vi "FeedbackDecode_UpdateDatabase.vi"(3 "DatabaseIn":T1={"ExperimentDate"=timestamp(3401556199.892892 s since 1904-01-01), "ImplantDate"=timestamp(3401890063 s since 1904-01-01), "CerebusFolder"="", "Experimenter"="Tyler Davis", "PatientNumber"="201102", "DominantHand"="Right", "DeviceType"="uECOG", "DeviceSerial"="CG-64BPX-F419", "DeviceHemisphere"="Right", "DeviceRegion"="Hand", "TaskType"="ArmMovementTask.vi", "TaskComments"="", "RecordingComments"="", "GeneralObservations"=""}, 4 "RecordsSelection":string="10/16/2011\u0000\u0000\u0000\u0000\u0000\u0000\u0000\u0000\u0000\u0000\u0000\u0000", 5 "CallType":enum16{"Initialize", "Save", "Load"}(ring)=enum."Load", 6 "DatabaseUDL":path=path "E:/Data/PatientDatabase.udl") -> (0 "DatabaseOut":T1={"ExperimentDate"=timestamp(3401556199.892892 s since 1904-01-01), "ImplantDate"=timestamp(3401890063 s since 1904-01-01), "CerebusFolder"="", "Experimenter"="Tyler Davis", "PatientNumber"="201102", "DominantHand"="Right", "DeviceType"="uECOG", "DeviceSerial"="CG-64BPX-F419", "DeviceHemisphere"="Right", "DeviceRegion"="Hand", "TaskType"="ArmMovementTask.vi", "TaskComments"="", "RecordingComments"="", "GeneralObservations"=""}, 1 "CerebusFoldersDates":string[](array[string]), 2 "ExperimentDatesSorted":string[](array[string]))   [LabVIEW 2020]
uses:
  <vilib>/addons/database/Connection.llb/DB Tools Open Connec (Path).vi
  <vilib>/addons/database/_DB Variant To Data/Database Variant To Data.xnode
  <vilib>/addons/database/NI_Database_API.lvlib
panel:
  out "ExperimentDates":string[](array[string])
  out "Fields":string[](array[string])=["ExperimentDate", "ImplantDate", "CerebusFolder", "Experimenter", "PatientNumber", "DominantHand", "DeviceType", "DeviceSerial", "DeviceHemisphere", "DeviceRegion", "TaskType", "TaskComments", "RecordingComments", "GeneralObservations"]
  # "Do not place ';' or '=' in the comment fields"
  # "Do not place ';' or '=' in the comment fields"
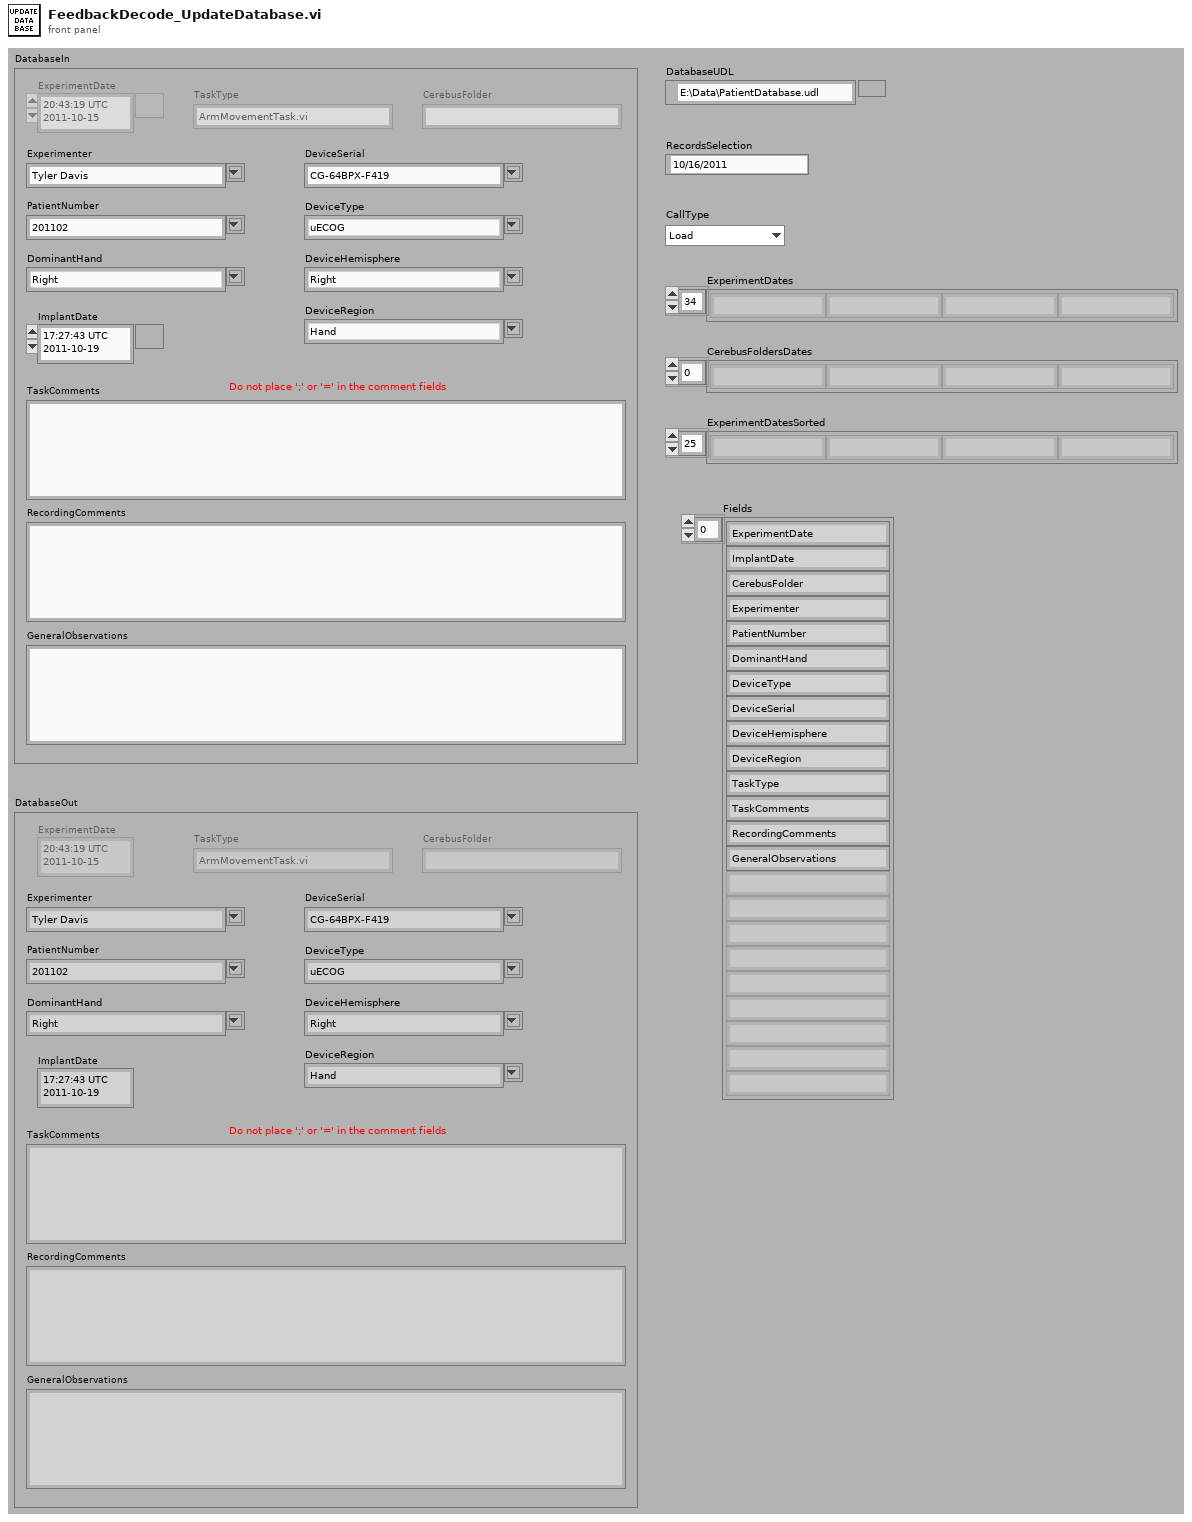
[diagram p1: front panel]
types:
  T1 = cluster{"ExperimentDate":timestamp, "ImplantDate":timestamp, "CerebusFolder":string, "Experimenter":string, "PatientNumber":string, "DominantHand":string, "DeviceType":string, "DeviceSerial":string, "DeviceHemisphere":string, "DeviceRegion":string, "TaskType":string, "TaskComments":string, "RecordingComments":string, "GeneralObservations":string}
  T2 = typedef "NI_Database_API.lvlib/Conn ObjectReference.ctl" = refnum<k1>
  T3 = cluster{"data":timestamp, "data":timestamp, "data":string, "data":string, "data":string, "data":string, "data":string, "data":string, "data":string, "data":string, "data":string, "data":string, "data":string, "data":string}
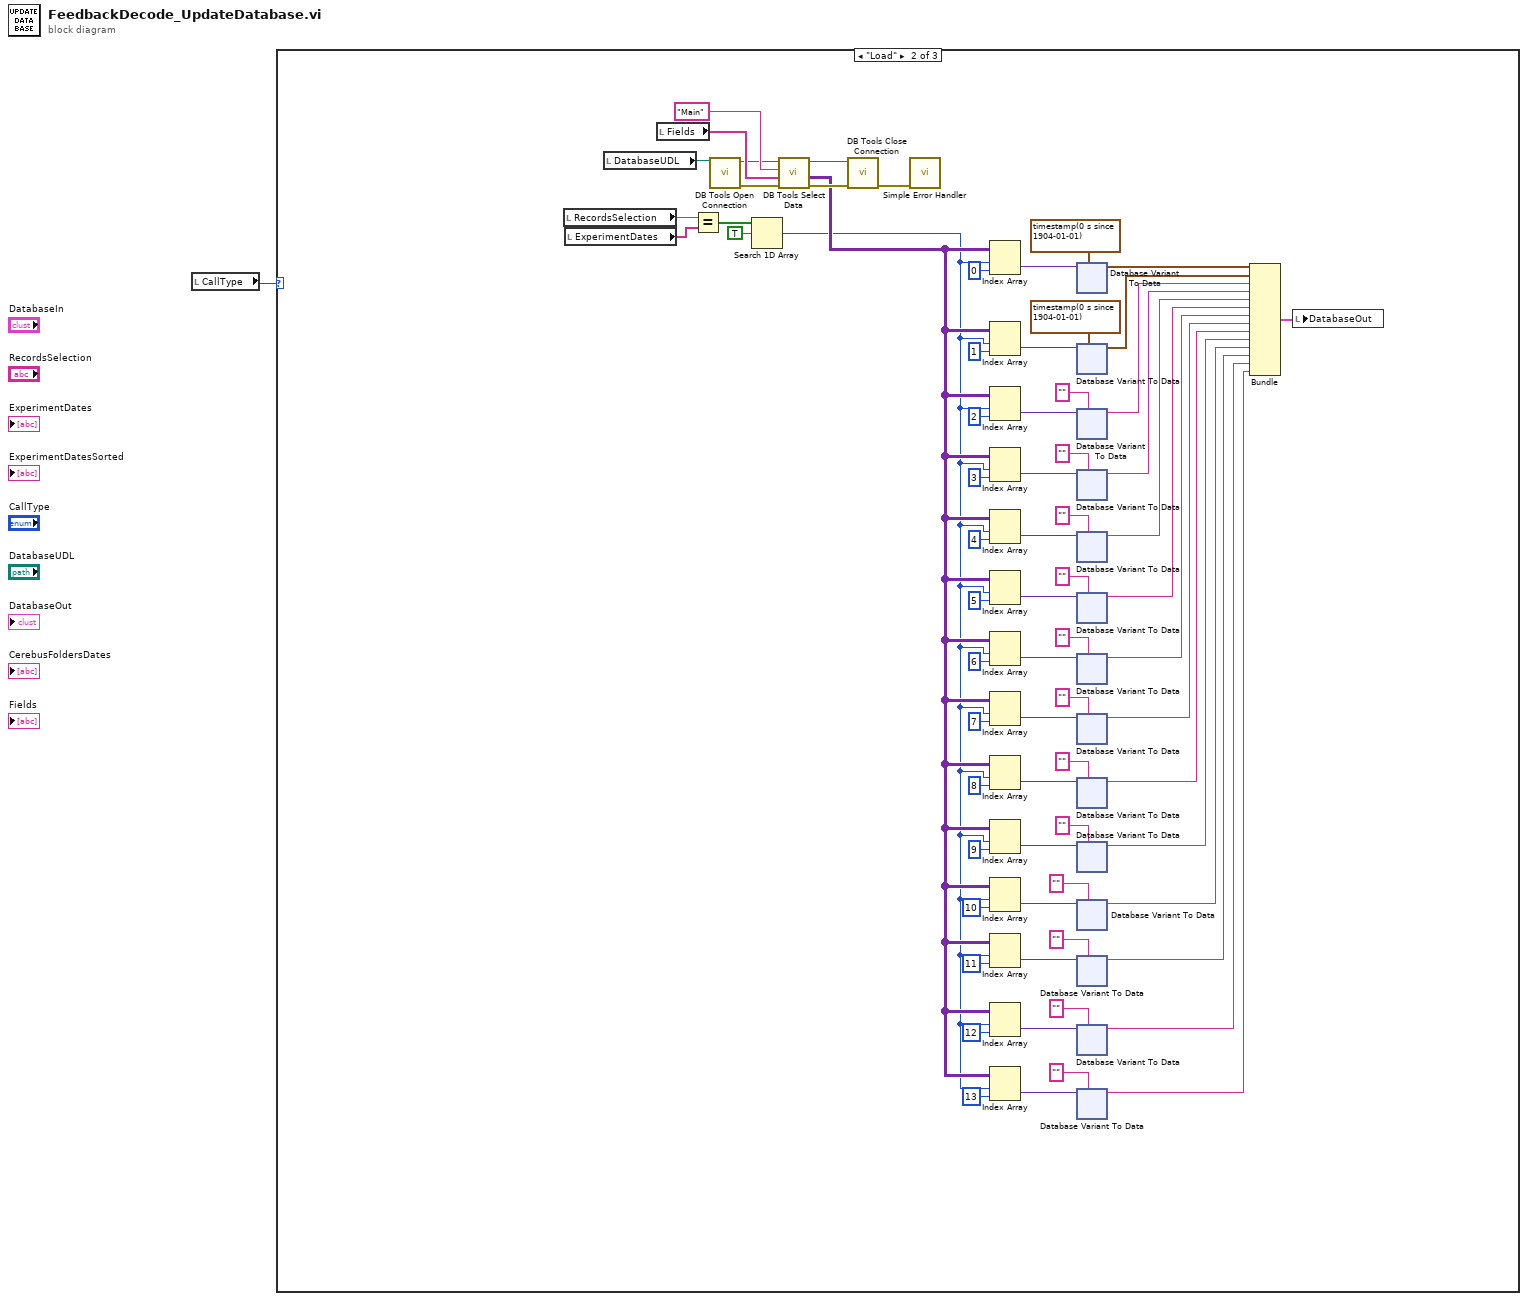
[diagram p0: block diagram]
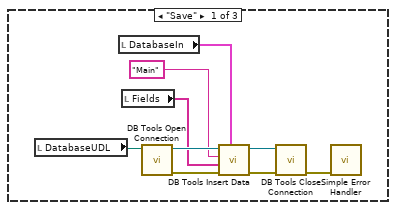
[diagram p2: hidden frame]
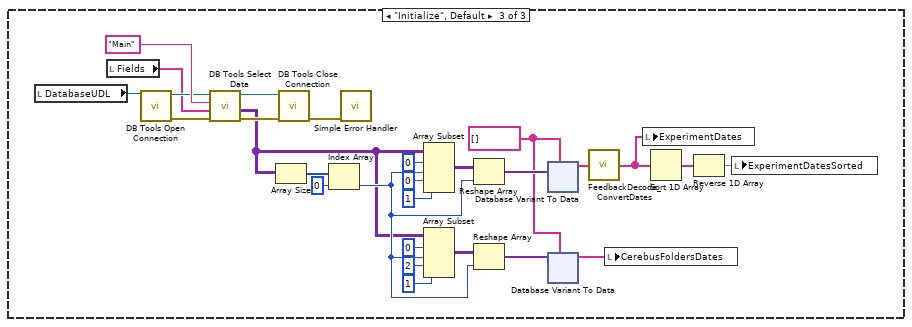
[diagram p3: hidden frame]
diagram:
  n1 = local read "CallType"() -> (w1:enum16{"Initialize", "Save", "Load"})
  n2 = case shown="\"Load\"" w1 {
    frame "Save" {
      n3 = local read "DatabaseUDL"() -> (w2:path)
      n4 = local read "DatabaseIn"() -> (w3:T1)
      n5 = local read "Fields"() -> (w4:string[])
      n6 = call-poly <vilib>:"DB Tools Open Connection.vi"("connection information"=w2) -> ("error out"=w8:errorcluster, "connection reference"=w10:T2)  [unwired: 7 in]
      n7 = call <vilib>:"DB Tools Insert Data.vi"("data"=w3, "error in (no error)"=w8, "columns"=w4, "table"="Main", "connection reference"=w10) -> ("error out"=w7:errorcluster, "connection reference out"=w6:T2)  [unwired: 5 in]
      n8 = call <vilib>:"DB Tools Close Connection.vi"("error in (no error)"=w7, "connection reference"=w6) -> ("error out"=w5:errorcluster)  [unwired: 5 in]
      n9 = call <vilib>:"Simple Error Handler.vi"("error in (no error)"=w5) -> ()  [unwired: 4 in, 5 out]
    }
    frame "Load" {
      n10 = local read "RecordsSelection"() -> (w32:string)
      n11 = local read "ExperimentDates"() -> (w31:string[])
      n12 = local read "DatabaseUDL"() -> (w79:path)
      n13 = local read "Fields"() -> (w77:string[])
      n14 = Equal?(x=w32, y=w31) -> (x = y?=w33:bool[])
      n15 = call-poly <vilib>:"DB Tools Open Connection.vi"("connection information"=w79) -> ("error out"=w81:errorcluster, "connection reference"=w74:T2)  [unwired: 7 in]
      n16 = Search 1D Array(1D array=w33, element=TRUE) -> (index of element=w11:i32)  [unwired: 1 in]
      n17 = call <vilib>:"DB Tools Select Data.vi"("error in (no error)"=w81, "columns"=w77, "table"="Main", "connection reference"=w74) -> ("error out"=w76:errorcluster, "data"=w13:variant[][], "connection reference out"=w75:T2)  [unwired: 2 in]
      n18 = call <vilib>:"DB Tools Close Connection.vi"("error in (no error)"=w76, "connection reference"=w75) -> ("error out"=w80:errorcluster)  [unwired: 5 in]
      n19 = call <vilib>:"Simple Error Handler.vi"("error in (no error)"=w80) -> ()  [unwired: 4 in, 5 out]
      n20 = Index Array(array=w13, index (row)=w11, index (col)=0 ("disabled index (col)")) -> (element=w72:variant)
      n21 = Index Array(array=w13, index (row)=w11, index (col)=1 ("disabled index (col)")) -> (element=w25:variant)
      n22 = Index Array(array=w13, index (row)=w11, index (col)=2 ("disabled index (col)")) -> (element=w70:variant)
      n23 = Index Array(array=w13, index (row)=w11, index (col)=3 ("disabled index (col)")) -> (element=w35:variant)
      n24 = Index Array(array=w13, index (row)=w11, index (col)=4 ("disabled index (col)")) -> (element=w65:variant)
      n25 = Index Array(array=w13, index (row)=w11, index (col)=5 ("disabled index (col)")) -> (element=w60:variant)
      n26 = Index Array(array=w13, index (row)=w11, index (col)=6 ("disabled index (col)")) -> (element=w59:variant)
      n27 = Index Array(array=w13, index (row)=w11, index (col)=7 ("disabled index (col)")) -> (element=w54:variant)
      n28 = Index Array(array=w13, index (row)=w11, index (col)=8 ("disabled index (col)")) -> (element=w53:variant)
      n29 = Index Array(array=w13, index (row)=w11, index (col)=9 ("disabled index (col)")) -> (element=w48:variant)
      n30 = Index Array(array=w13, index (row)=w11, index (col)=10 ("disabled index (col)")) -> (element=w47:variant)
      n31 = Index Array(array=w13, index (row)=w11, index (col)=11 ("disabled index (col)")) -> (element=w27:variant)
      n32 = Index Array(array=w13, index (row)=w11, index (col)=12 ("disabled index (col)")) -> (element=w21:variant)
      n33 = Index Array(array=w13, index (row)=w11, index (col)=13 ("disabled index (col)")) -> (element=w14:variant)
      n34 = xnode "Database Variant To Data"("database variant"=w72, "type"=timestamp(0 s since 1904-01-01)) -> ("data"=w26:timestamp)  [unwired: 1 in, 1 out]
      n35 = xnode "Database Variant To Data"("database variant"=w25, "type"=timestamp(0 s since 1904-01-01)) -> ("data"=w23:timestamp)  [unwired: 1 in, 1 out]
      n36 = xnode "Database Variant To Data"("database variant"=w70, "type"="") -> ("data"=w45:string)  [unwired: 1 in, 1 out]
      n37 = xnode "Database Variant To Data"("database variant"=w35, "type"="") -> ("data"=w44:string)  [unwired: 1 in, 1 out]
      n38 = xnode "Database Variant To Data"("database variant"=w65, "type"="") -> ("data"=w43:string)  [unwired: 1 in, 1 out]
      n39 = xnode "Database Variant To Data"("database variant"=w60, "type"="") -> ("data"=w42:string)  [unwired: 1 in, 1 out]
      n40 = xnode "Database Variant To Data"("database variant"=w59, "type"="") -> ("data"=w41:string)  [unwired: 1 in, 1 out]
      n41 = xnode "Database Variant To Data"("database variant"=w54, "type"="") -> ("data"=w40:string)  [unwired: 1 in, 1 out]
      n42 = xnode "Database Variant To Data"("database variant"=w53, "type"="") -> ("data"=w39:string)  [unwired: 1 in, 1 out]
      n43 = xnode "Database Variant To Data"("database variant"=w48, "type"="") -> ("data"=w38:string)  [unwired: 1 in, 1 out]
      n44 = xnode "Database Variant To Data"("database variant"=w47, "type"="") -> ("data"=w37:string)  [unwired: 1 in, 1 out]
      n45 = xnode "Database Variant To Data"("database variant"=w27, "type"="") -> ("data"=w28:string)  [unwired: 1 in, 1 out]
      n46 = xnode "Database Variant To Data"("database variant"=w21, "type"="") -> ("data"=w18:string)  [unwired: 1 in, 1 out]
      n47 = xnode "Database Variant To Data"("database variant"=w14, "type"="") -> ("data"=w12:string)  [unwired: 1 in, 1 out]
      n48 = Bundle("data"=w26, "data"=w23, "data"=w45, "data"=w44, "data"=w43, "data"=w42, "data"=w41, "data"=w40, "data"=w39, "data"=w38, "data"=w37, "data"=w28, "data"=w18, "data"=w12) -> (w17:T3)  [unwired: 1 in]
      n49 = local write "DatabaseOut"(w17) -> ()
    }
    frame "Initialize", Default {
      w563 = string[] []
      n50 = local read "DatabaseUDL"() -> (w581:path)
      n51 = local read "Fields"() -> (w569:string[])
      n52 = call-poly <vilib>:"DB Tools Open Connection.vi"("connection information"=w581) -> ("error out"=w583:errorcluster, "connection reference"=w577:T2)  [unwired: 7 in]
      n53 = call <vilib>:"DB Tools Select Data.vi"("error in (no error)"=w583, "columns"=w569, "table"="Main", "connection reference"=w577) -> ("error out"=w579:errorcluster, "data"=w561:variant[][], "connection reference out"=w578:T2)  [unwired: 2 in]
      n54 = Array Size(array=w561) -> (size(s)=w575:i32[])
      n55 = call <vilib>:"DB Tools Close Connection.vi"("error in (no error)"=w579, "connection reference"=w578) -> ("error out"=w582:errorcluster)  [unwired: 5 in]
      n56 = Index Array(array=w575, index=0) -> (element=w564:i32)
      n57 = call <vilib>:"Simple Error Handler.vi"("error in (no error)"=w582) -> ()  [unwired: 4 in, 5 out]
      n58 = Array Subset(array=w561, index (row)=0 ("index"), length (row)=w564, index (col)=0 ("index"), length (col)=1 ("length")) -> (w571:variant[][])
      n59 = Array Subset(array=w561, index (row)=0 ("index"), length (row)=w564, index (col)=2 ("index"), length (col)=1 ("length")) -> (w568:variant[][])
      n60 = Reshape Array(w571, w564) -> (w570:variant[])
      n61 = Reshape Array(w568, w564) -> (w562:variant[])
      n62 = xnode "Database Variant To Data"("database variant"=w570, "type"=w563) -> ("data"=w557:string[])  [unwired: 1 in, 1 out]
      n63 = xnode "Database Variant To Data"("database variant"=w562, "type"=w563) -> ("data"=w560:string[])  [unwired: 1 in, 1 out]
      n64 = call "FeedbackDecode_ConvertDates.vi"("Dates"=w557) -> ("ConvertedDates"=w556:string[])
      n65 = local write "CerebusFoldersDates"(w560) -> ()
      n66 = local write "ExperimentDates"(w556) -> ()
      n67 = Sort 1D Array(array=w556) -> (sorted array=w559:string[])
      n68 = Reverse 1D Array(array=w559) -> (reversed array=w558:string[])
      n69 = local write "ExperimentDatesSorted"(w558) -> ()
    }
  }
